vi "Calculate_1.vi"(11 "Operators":string[](array[string])) -> (2 "Value Out":u64, 3 "Operators Out":string[](array[string]))   [LabVIEW 2018]
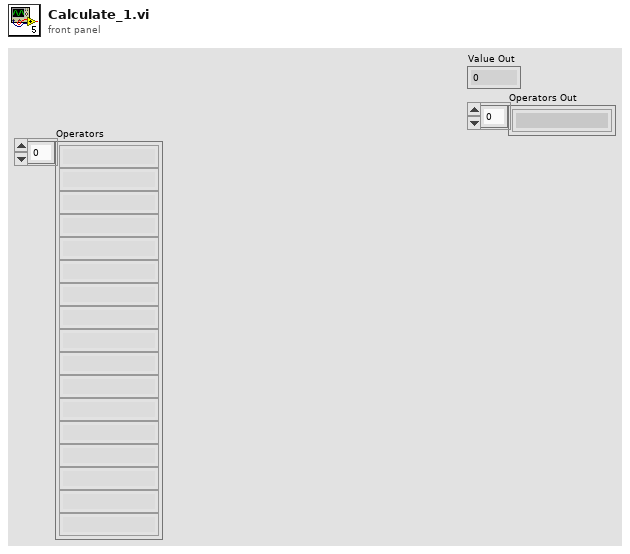
[diagram p1: front panel]
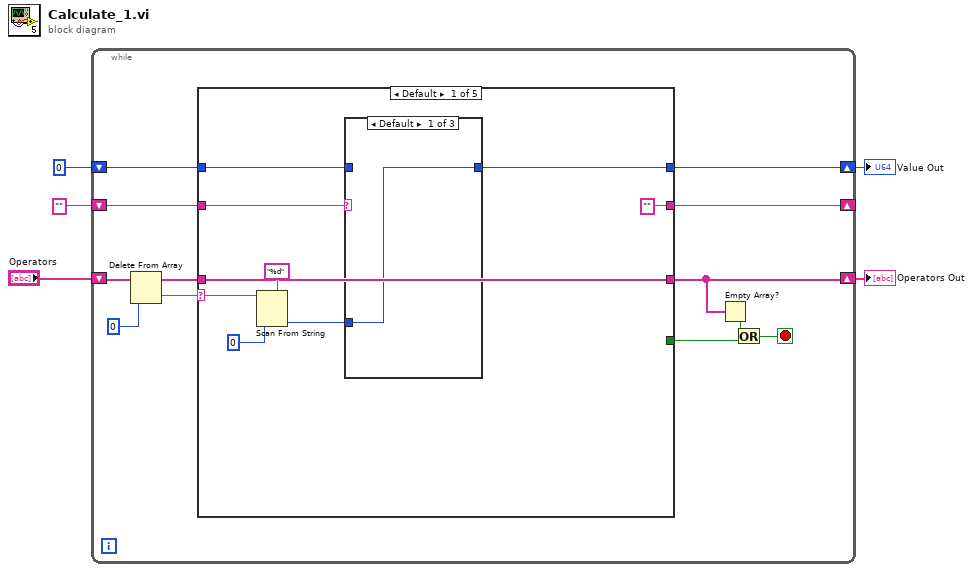
[diagram p0: block diagram]
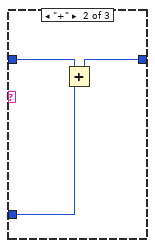
[diagram p2: hidden frame]
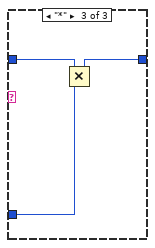
[diagram p3: hidden frame]
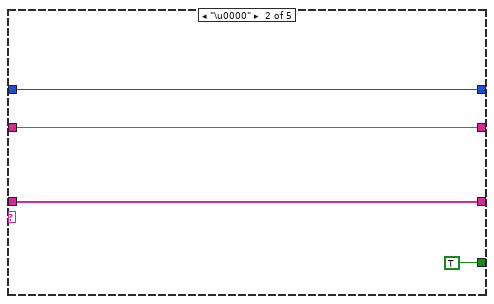
[diagram p4: hidden frame]
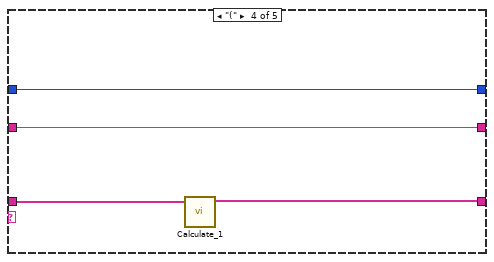
[diagram p6: hidden frame]
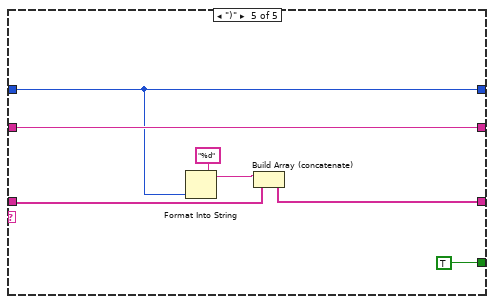
[diagram p7: hidden frame]
diagram:
  n1 = while {
    shift-right: [w15] -> w2
    shift-left: u64 0 -> [w14]
    shift-right: [w17] -> _
    shift-left: "" -> [w16]
    shift-right: [w9] -> w1
    shift-left: "Operators" -> [w13]
    stop <- w7 stop-if-true
    n2 = Delete From Array(array=w13, index=0) -> (deleted portion=w11:string, array with subset deleted=w10:string[])  [unwired: 1 in]
    n3 = case shown="Default" w11 {
      selector: w11 -> [w23 _ w39 _ _]
      tunnel: ["" w35 w39 w41 w51] -> w17
      tunnel: w16 -> [w26 w35 _ w41 w51]
      tunnel: [w20 w34 w40 w42 w50] -> w15
      tunnel: w14 -> [w25 w34 w40 w42 w50]
      tunnel: w10 -> [w18 w36 w38 w44 w47]
      tunnel: [w18 w36 w38 w43 w46] -> w9
      tunnel: [_ TRUE _ _ TRUE] -> w6
      frame Default {
        n4 = Scan From String(format string="%d", input string=w23, default 1=u64 0) -> (output 1=w21:u64)  [unwired: 2 in, 3 out]
        n5 = case shown="Default" w26 {
          tunnel: w25 -> [_ w30 w33]
          tunnel: w21 -> [w27 w29 w32]
          tunnel: [w27 w28 w31] -> w20
          frame Default {
          }
          frame "+" {
            n6 = Add(x=w30, y=w29) -> (x+y=w28:u64)
          }
          frame "*" {
            n7 = Multiply(x=w33, y=w32) -> (x*y=w31:u64)
          }
        }
      }
      frame "\u0000" {
      }
      frame "*", "+" {
      }
      frame "(" {
        n8 = call "Calculate_1.vi"("Operators"=w44) -> ("Operators Out"=w43:string[])  [unwired: 9 in, 1 out]
      }
      frame ")" {
        n9 = Format Into String(format string="%d", w50) -> (resulting string=w48:string)  [unwired: 2 in, 1 out]
        n10 = Build Array (concatenate)(w48, w47) -> (w46:string[])
      }
    }
    n11 = Empty Array?(array=w9) -> (empty?=w8:bool)
    n12 = Or(x=w8, y=w6) -> (x .or. y?=w7:bool)
  }
  "Value Out" <- w2
  "Operators Out" <- w1
